vi "CalculateAngle (SubVI).vi"(11 "axis info":T1) -> (3 "Angle [°]":dbl)   [LabVIEW 2015]
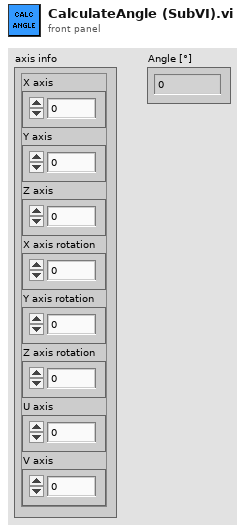
[diagram p1: front panel]
types:
  T1 = cluster{"X axis":i32, "Y axis":i32, "Z axis":i32, "X axis rotation":i32, "Y axis rotation":i32, "Z axis rotation":i32, "U axis":i32, "V axis":i32}
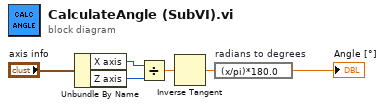
[diagram p0: block diagram]
diagram:
  n1 = Unbundle By Name("axis info") -> ("X axis"=w4:i32, "Z axis"=w5:i32)
  n2 = Divide(x=w4, y=w5) -> (x/y=w2:dbl)
  n3 = Inverse Tangent(1:w2) -> (0:w3:dbl)
  n4 = expression code="(x/pi)*180.0" "radians to degrees"(w3) -> (→"Angle [°]":dbl)
